vi "Write value as Boolean.vi"(8 "error in (no error)":errorcluster, 10 "value":bool, 11 "JSON String in":refnum<class "JSON Helper.lvclass">) -> (0 "error out":errorcluster, 3 "JSON String out":refnum<class "JSON Helper.lvclass">)   [LabVIEW 2016, in "JSON Helper.lvclass"]
uses:
  JSON Helper/JSON Helper.lvclass
  JSON Helper/JSON Helper.lvclass/JSON Helper.ctl
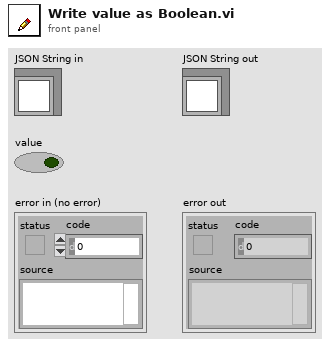
[diagram p1: front panel]
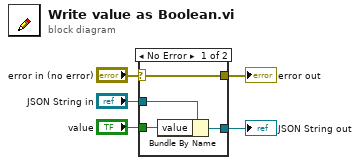
[diagram p0: block diagram]
diagram:
  n1 = case shown="No Error" "error in (no error)" {
    selector: "error in (no error)" -> [w9 w10]
    tunnel: [w9 w10] -> w4
    tunnel: [w7 w11] -> w2
    tunnel: "JSON String in" -> [w8 w11]
    tunnel: "value" -> [w6 _]
    frame No Error {
      n2 = Bundle By Name(cluster=w8, "value"=w6) -> (w7:refnum<class "JSON Helper.lvclass">)
    }
    frame Error {
    }
  }
  "error out" <- w4
  "JSON String out" <- w2
